vi "LookupWord.vi"(8 "error in (no error)":errorcluster, 10 "Word":string) -> (0 "error out":errorcluster, 1 "Result":T1, 2 "Exists?":bool)   [LabVIEW 2024, in "GUI.lvlib" / "Controller.lvclass"]
uses:
  Controller.lvclass
  Controller.lvclass/Controller.ctl
  <vilib>/httpClient/LabVIEWHTTPClient.lvlib
  TypeDefs/LookupResult.ctl
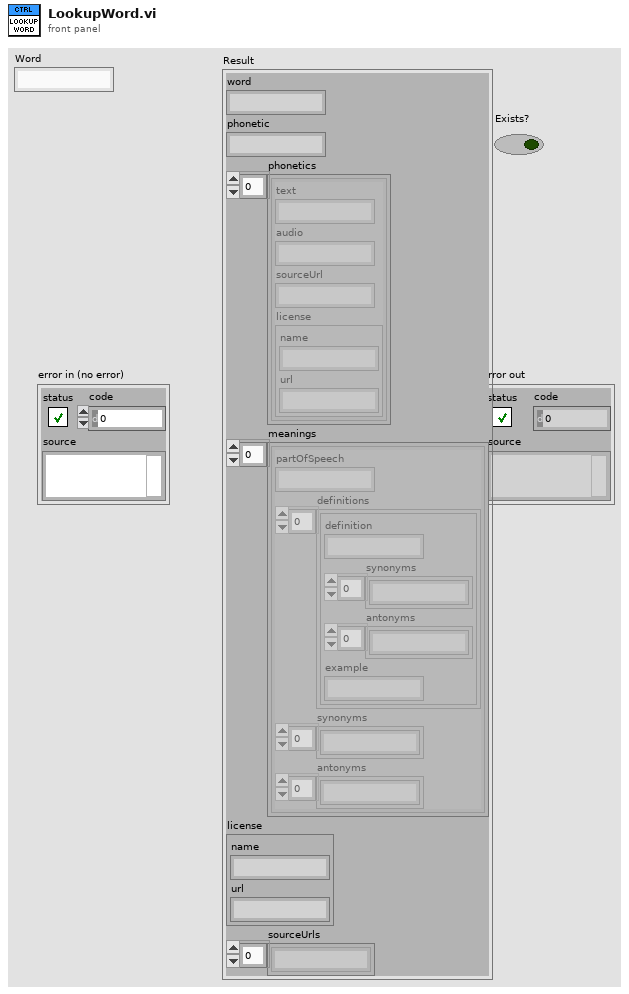
[diagram p1: front panel]
types:
  T1 = cluster{"word":string, "phonetic":string, "phonetics":cluster{"text":string, "audio":string, "sourceUrl":string, "license":cluster{"name":string, "url":string}}[], "meanings":cluster{"partOfSpeech":string, "definitions":cluster{"definition":string, "synonyms":string[], "antonyms":string[], "example":string}[], "synonyms":string[], "antonyms":string[]}[], "license":cluster{"name":string, "url":string}, "sourceUrls":string[]}
  T2 = typedef "LookupResult.ctl" = cluster{"word":string, "phonetic":string, "phonetics":cluster{"text":string, "audio":string, "sourceUrl":string, "license":cluster{"name":string, "url":string}}[], "meanings":cluster{"partOfSpeech":string, "definitions":cluster{"definition":string, "synonyms":string[], "antonyms":string[], "example":string}[], "synonyms":string[], "antonyms":string[]}[], "license":cluster{"name":string, "url":string}, "sourceUrls":string[]}
  T3 = cluster{"title":string, "message":string, "resolution":string}
  T4 = typedef "LabVIEWHTTPClient.lvlib/ClientHandle.ctl" = refnum<k1>
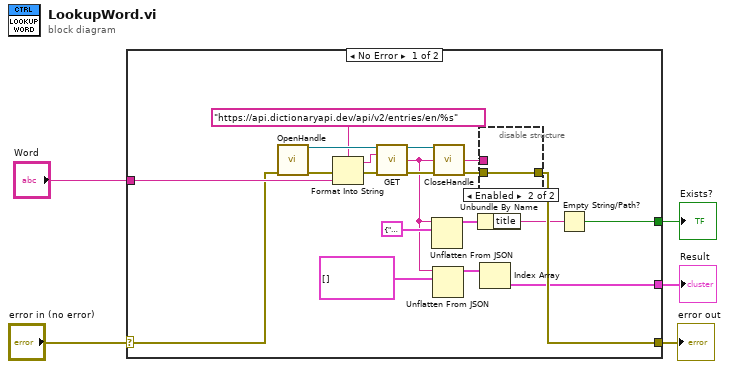
[diagram p0: block diagram]
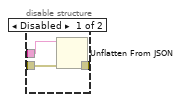
[diagram p2: hidden frame]
diagram:
  n1 = case shown="No Error" "error in (no error)" {
    selector: "error in (no error)" -> [w15 w29]
    tunnel: [w14 w29] -> w4
    tunnel: "Word" -> [w17 _]
    tunnel: [w7 _] -> w2
    tunnel: [w6 _] -> w1
    frame No Error {
      n2 = call <vilib>:"OpenHandle.vi"("error in (no error)"=w15) -> ("client handle out"=w24:T4, "error out"=w20:errorcluster)  [unwired: 13 in]
      n3 = Format Into String(format string="https://api.dictionaryapi.dev/api/v2/entries/en/%s" ("url"), error in=w20, w17) -> (resulting string=w18:string, error out=w19:errorcluster)  [unwired: 1 in]
      n4 = call <vilib>:"GET.vi"("client handle"=w24, "url"=w18, "error in (no error)"=w19) -> ("client handle out"=w23:T4, "body"=w12:string, "error out"=w22:errorcluster)  [unwired: 9 in, 1 out]
      n5 = Unflatten From JSON(JSON string=w12, type and defaults=T3 {"title"="", "message"="", "resolution"=""}) -> (value=w10:T3)  [unwired: 5 in, 1 out]
      n6 = Unflatten From JSON(JSON string=w12, type and defaults=T2[] []) -> (value=w9:T2[])  [unwired: 5 in, 1 out]
      n7 = call <vilib>:"CloseHandle.vi"("client handle"=w23, "error in (no error)"=w22) -> ("error out"=w16:errorcluster)  [unwired: 13 in]
      n8 = Unbundle By Name(w10) -> ("title"=w8:string)
      n9 = disable-structure shown="Enabled" {
        disable-tunnel: w12 -> [w27 _]
        disable-tunnel: w16 -> [w26 w28]
        disable-tunnel: [w25 w28] -> w14
        frame Disabled {
          n10 = Unflatten From JSON(JSON string=w27, error in (no error)=w26) -> (error out=w25:errorcluster)  [unwired: 5 in, 1 out]
        }
        frame Enabled {
        }
      }
      n11 = Index Array(array=w9) -> (element=w6:T2)  [unwired: 1 in]
      n12 = Empty String/Path?(string/path=w8) -> (empty?=w7:bool)
    }
    frame Error {
    }
  }
  "error out" <- w4
  "Exists?" <- w2
  "Result" <- w1
